vi "angle_mag.vi"(8 "x":dbl(slide) scale=0.0..10.0, 11 "y":dbl(slide) scale=0.0..10.0) -> (0 "mag":dbl, 3 "angle":dbl)   [LabVIEW 2023]
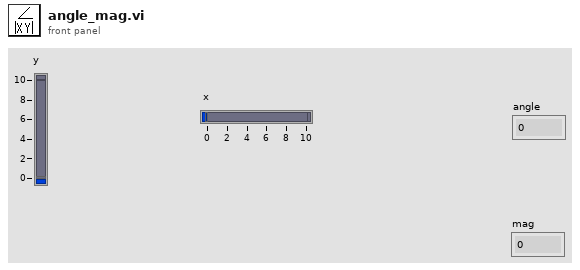
[diagram p1: front panel]
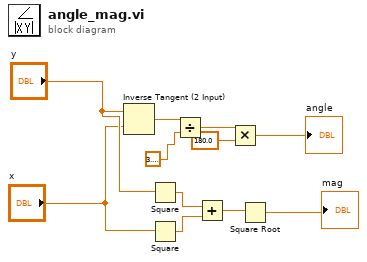
[diagram p0: block diagram]
diagram:
  n1 = Inverse Tangent (2 Input)(1:"x", 2:"y") -> (0:w11:dbl)
  n2 = Square(x="y") -> (x^2=w7:dbl)
  n3 = Square(x="x") -> (x^2=w6:dbl)
  n4 = Divide(x=w11, y=3.141592653589793) -> (x/y=w9:dbl)
  n5 = Add(x=w7, y=w6) -> (x+y=w5:dbl)
  n6 = Multiply(x=w9, y=180.0) -> (x*y=→"angle":dbl)
  n7 = Square Root(x=w5) -> (sqrt(x)=→"mag":dbl)
